vi "finish5RobotsPassGamePlay.vi"(8 "error in (no error)":errorcluster, 10 "Game in":refnum<class "Game.lvclass">, 11 "5RobotsPassGamePlay in":refnum<class "5RobotsPassGamePlay.lvclass">) -> (0 "error out":errorcluster, 1 "finish?":bool, 2 "Game out":refnum<class "Game.lvclass">, 3 "5RobotsPassGamePlay out":refnum<class "5RobotsPassGamePlay.lvclass">, 4 "debugOffensivePlayFinished":T1[](array[typedef]), 5 "degugBallVel":T2[](array[typedef]))   [LabVIEW 2020, in "5RobotsPassGamePlay.lvclass"]
uses:
  5RobotsPassGamePlay.lvclass
  C:/RoboIME/SSL_AI/Play_class/Play.lvclass
  Game_class/Game.lvclass
  PassFinishBallVelConditionDegub.ctl
  PassFinishReceiverDistanceToBallConditionDebug.ctl
  Referee_class/command_interpreted.ctl
  Utilities_class/Utilities.lvclass
  Robot_class/roles.ctl
  Game_class/Game.lvclass/Game.ctl
  Events_class/Events.lvclass/Events.ctl
  Object_class/Object.lvclass/Object.ctl
  Ball_class/Ball.lvclass/Ball.ctl
  Parameters_class/Parameters.lvclass/Parameters.ctl
  Referee_class/Referee.lvclass/Referee.ctl
  Team_class/Team.lvclass/Team.ctl
  Robot_class/Robot.lvclass/Robot.ctl
  Playbook_class/Playbook.lvclass/Playbook.ctl
  5RobotsPassGamePlay.lvclass/5RobotsPassGamePlay.ctl
  Playbook_class/Read offensive_plays.vi
  Write factorPassAlreadyCalculated_.vi
  Write passFinishConditions.vi
  Playbook_class/Write offensive_plays.vi
  Game_class/Read Parameters.lvclass.vi
  Parameters_class/Read BallVelToAbortPass.vi
  Parameters_class/Read minDistanceToPass.vi
  Game_class/Read EventsRef.vi
  Game_class/Read BallRef.vi
  Game_class/Read OffensiveTeam.vi
  Team_class/Read RobotRef.vi
  Team_class/Read OffensivePlay Finished.vi
  Object_class/Read x.vi
  Object_class/Read y.vi
  Robot_class/Read id.vi
  Ball_class/Read z.vi
  Ball_class/Read v_x.vi
  Ball_class/Read v_y.vi
  Events_class/Read touch.vi
  Events_class/Read enemy_ball_possesion.vi
  Events_class/Read id_touch.vi
  Events_class/Read ball_out.vi
  Game_class/Read Referee.vi
  Referee_class/Read command_interpreted.vi
  Ally_class/Ally.lvclass
  C:/RoboIME/SSL_AI/Team_class/Team.lvclass
  Robot_class/Robot.lvclass
  C:/RoboIME/SSL_AI/Object_class/Object.lvclass
  Ball_class/Ball.lvclass
  Referee_class/Referee.lvclass
  Events_class/Events.lvclass
  Parameters_class/Parameters.lvclass
  Playbook_class/Playbook.lvclass
  Play_class/Play.lvclass
  TestPlay_class/TestPlay.lvclass
  EnemyPossessionAtEnemyFieldPlay_class/EnemyPossessionAtEnemyFieldPlay.lvclass
  EnemyPossessionAtOurFieldPlay_class/EnemyPossessionAtOurFieldPlay.lvclass
  NormalGamePlay_class/NormalGamePlay.lvclass
  IndirectEnemyPlay_class/IndirectEnemyPlay.lvclass
  PrepareKickoffAllyPlay_class/PrepareKickoffAllyPlay.lvclass
  PrepareKickoffEnemyPlay_class/PrepareKickoffEnemyPlay.lvclass
  KickPenaltyAllyPlay_class/KickPenaltyAllyPlay.lvclass
  PreparePenaltyAllyPlay_class/PreparePenaltyAllyPlay.lvclass
  DirectEnemyPlay_class/DirectEnemyPlay.lvclass
  PreparePenaltyEnemyPlay_class/PreparePenaltyEnemyPlay.lvclass
  BallOutOfFieldPlay_class/BallOutOfFieldPlay.lvclass
  StopOffensivePlay_class/StopOffensivePlay.lvclass
  PassPlay_class/PassPlay.lvclass
  DirectKickPlay_class/DirectKickPlay.lvclass
  HaltPlay_class/HaltPlay.lvclass
  PreparePassPlay_class/PreparePassPlay.lvclass
  PassToStriker_class/PassToStriker.lvclass
  PassTo2ndStriker_class/PassTo2ndStriker.lvclass
  SimplePass_class/SimplePass.lvclass
  PrepareRollToPassPlay_class/PrepareRollToPassPlay.lvclass
  PrepareDoublePassPlay_class/PrepareDoublePassPlay.lvclass
  TableWith2ndStrikerPlay_class/TableWith2ndStrikerPlay.lvclass
  TableWithStrikerPlay_class/TableWithStrikerPlay.lvclass
  PrepareTriplePassPlay_class/PrepareTriplePassPlay.lvclass
  ABCPassPlay_class/ABCPassPlay.lvclass
  PreparePassInGame1_class/PreparePassInGame1.lvclass
  ACBPassPlay_class/ACBPassPlay.lvclass
  PrepareKeeperPassPlay_class/PrepareKeeperPassPlay.lvclass
  KeeperPassToStrikerPlay_class/KeeperPassToStrikerPlay.lvclass
  5RobotsNormalGamePlay_class/5RobotsNormalGamePlay.lvclass
  5RobotsKeeperGame_class/5RobotsKeeperGame.lvclass
panel:
  in  "ReceiverDistanceToBallConditionDebug":T1
  in  "BallVelConditionDebug":T2
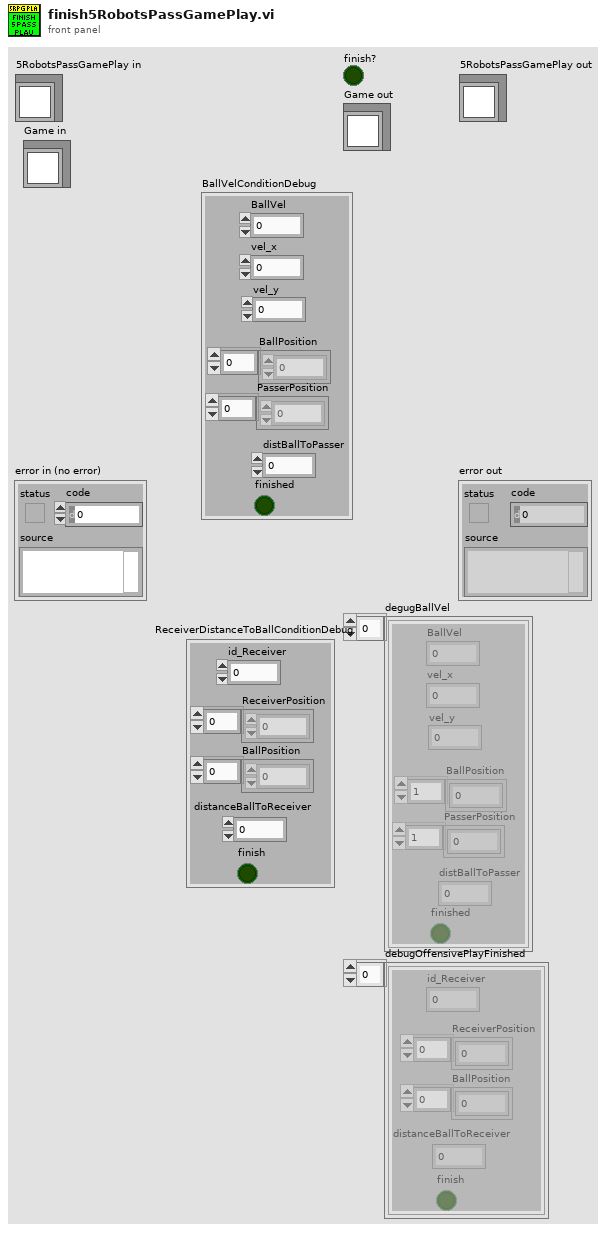
[diagram p1: front panel]
types:
  T1 = typedef "PassFinishReceiverDistanceToBallConditionDebug.ctl" = cluster{"id_Receiver":i32, "ReceiverPosition":dbl[], "BallPosition":dbl[], "distanceBallToReceiver":dbl, "finish":bool}
  T2 = typedef "PassFinishBallVelConditionDegub.ctl" = cluster{"BallVel":dbl, "BallPosition":dbl[], "PasserPosition":dbl[], "distBallToPasser":dbl, "finished":bool, "vel_x":dbl, "vel_y":dbl}
  T3 = typedef "roles.ctl" = enum16{"SecondMarker", "5Robots5th", "PassBestReceiver", "5Robots4th", "5Robots3rd", "5Robots2nd", "5Robots1st", "PassBestRobot", "WaitPass", "ABCThirdKicker", "ABCFirstKicker", "ABCSecondKicker", "Tabler", "TableFinalizer", "PrepareRollToPassRoller", "PrepareRollToPassReceiver", "SimplePassRoll", "SimplePassRollReceiver", "PenaltyDefense", "PreparePassReceiver 2", "PreparePassReceiver 1", "PassObserver", "Timeout", "Goto", "ZigZag", "None", "BallOutOfField", "DefenderArea", "Duelist", "AttackerStop", "FollowAttacker", "KeeperRole", "KickPenalty", "AttackerAimGoal", "AttackerBlock", "Marker", "Halt", "Shoot", "PassKicker", "PassReceiver", "TestRole", "PenaltyAttacker"}
  T4 = typedef "command_interpreted.ctl" = enum16{"Goal Ally", "Goal Enemy", "Ball Placement Enemy", "Ball Placement Ally", "Normal Half Time", "Extra Time  Break", "Extra Half Time", "None", "Post Game", "PKA Normal Start", "Prepare Kickoff Ally", "PKE Normal Start", "Prepare Kickoff Enemy", "Force Start", "Halt", "Timeout", "Prepare Penalty Ally", "Prepare Penalty Enemy", "PPA NormalStart", "PPE Normal Start", "Indirect Free Ally", "Direct Free Enemy", "Direct Free Ally", "Indirect Free Enemy", "Stop"}
  T5 = typedef "offensive_plays.ctl" = cluster{"Play":refnum<class "Play.lvclass">, "TestPlay":refnum<class "TestPlay.lvclass">, "EnemyPossessionAtEnemyFieldPlay":refnum<class "EnemyPossessionAtEnemyFieldPlay.lvclass">, "EnemyPossessionAtOurFieldPlay":refnum<class "EnemyPossessionAtOurFieldPlay.lvclass">, "NormalGamePlay":refnum<class "NormalGamePlay.lvclass">, "IndirectEnemyPlay":refnum<class "IndirectEnemyPlay.lvclass">, "PrepareKickoffAllyPlay":refnum<class "PrepareKickoffAllyPlay.lvclass">, "PrepareKickoffEnemyPlay":refnum<class "PrepareKickoffEnemyPlay.lvclass">, "KickPenaltyAllyPlay":refnum<class "KickPenaltyAllyPlay.lvclass">, "PreparePenaltyAllyPlay":refnum<class "PreparePenaltyAllyPlay.lvclass">, "DirectEnemyPlay":refnum<class "DirectEnemyPlay.lvclass">, "PreparePenaltyEnemyPlay":refnum<class "PreparePenaltyEnemyPlay.lvclass">, "BallOutOfFieldPlay":refnum<class "BallOutOfFieldPlay.lvclass">, "StopOffensivePlay":refnum<class "StopOffensivePlay.lvclass">, "PassPlay":refnum<class "PassPlay.lvclass">, "DirectKickPlay":refnum<class "DirectKickPlay.lvclass">, "HaltPlay":refnum<class "HaltPlay.lvclass">, "PreparePassPlay":refnum<class "PreparePassPlay.lvclass">, "PassToStrikerPlay":refnum<class "PassToStriker.lvclass">, "PassTo2ndStrikerPlay":refnum<class "PassTo2ndStriker.lvclass">, "SimplePassPlay":refnum<class "SimplePass.lvclass">, "PrepareRollToPassPlay":refnum<class "PrepareRollToPassPlay.lvclass">, "PrepareDoublePassPlay":refnum<class "PrepareDoublePassPlay.lvclass">, "TableWith2ndStrikerPlay":refnum<class "TableWith2ndStrikerPlay.lvclass">, "TableWithStrikerPlay":refnum<class "TableWithStrikerPlay.lvclass">, "PrepareTriplePassPlay":refnum<class "PrepareTriplePassPlay.lvclass">, "ABCPassPlay":refnum<class "ABCPassPlay.lvclass">, "PreparePassInGame1":refnum<class "PreparePassInGame1.lvclass">, "ACBPassPlay":refnum<class "ACBPassPlay.lvclass">, "PrepareKeeperPassPlay":refnum<class "PrepareKeeperPassPlay.lvclass">, "KeeperPassToStrikerPlay":refnum<class "KeeperPassToStrikerPlay.lvclass">, "SimplePass":refnum<class "SimplePass.lvclass">, "SimplePass 2":refnum<class "SimplePass.lvclass">, "5RobotsNormalGamePlay":refnum<class "5RobotsNormalGamePlay.lvclass">, "5RobotsPassGamePlay":refnum<class "5RobotsPassGamePlay.lvclass">, "5RobotsKeeperGame":refnum<class "5RobotsKeeperGame.lvclass">}
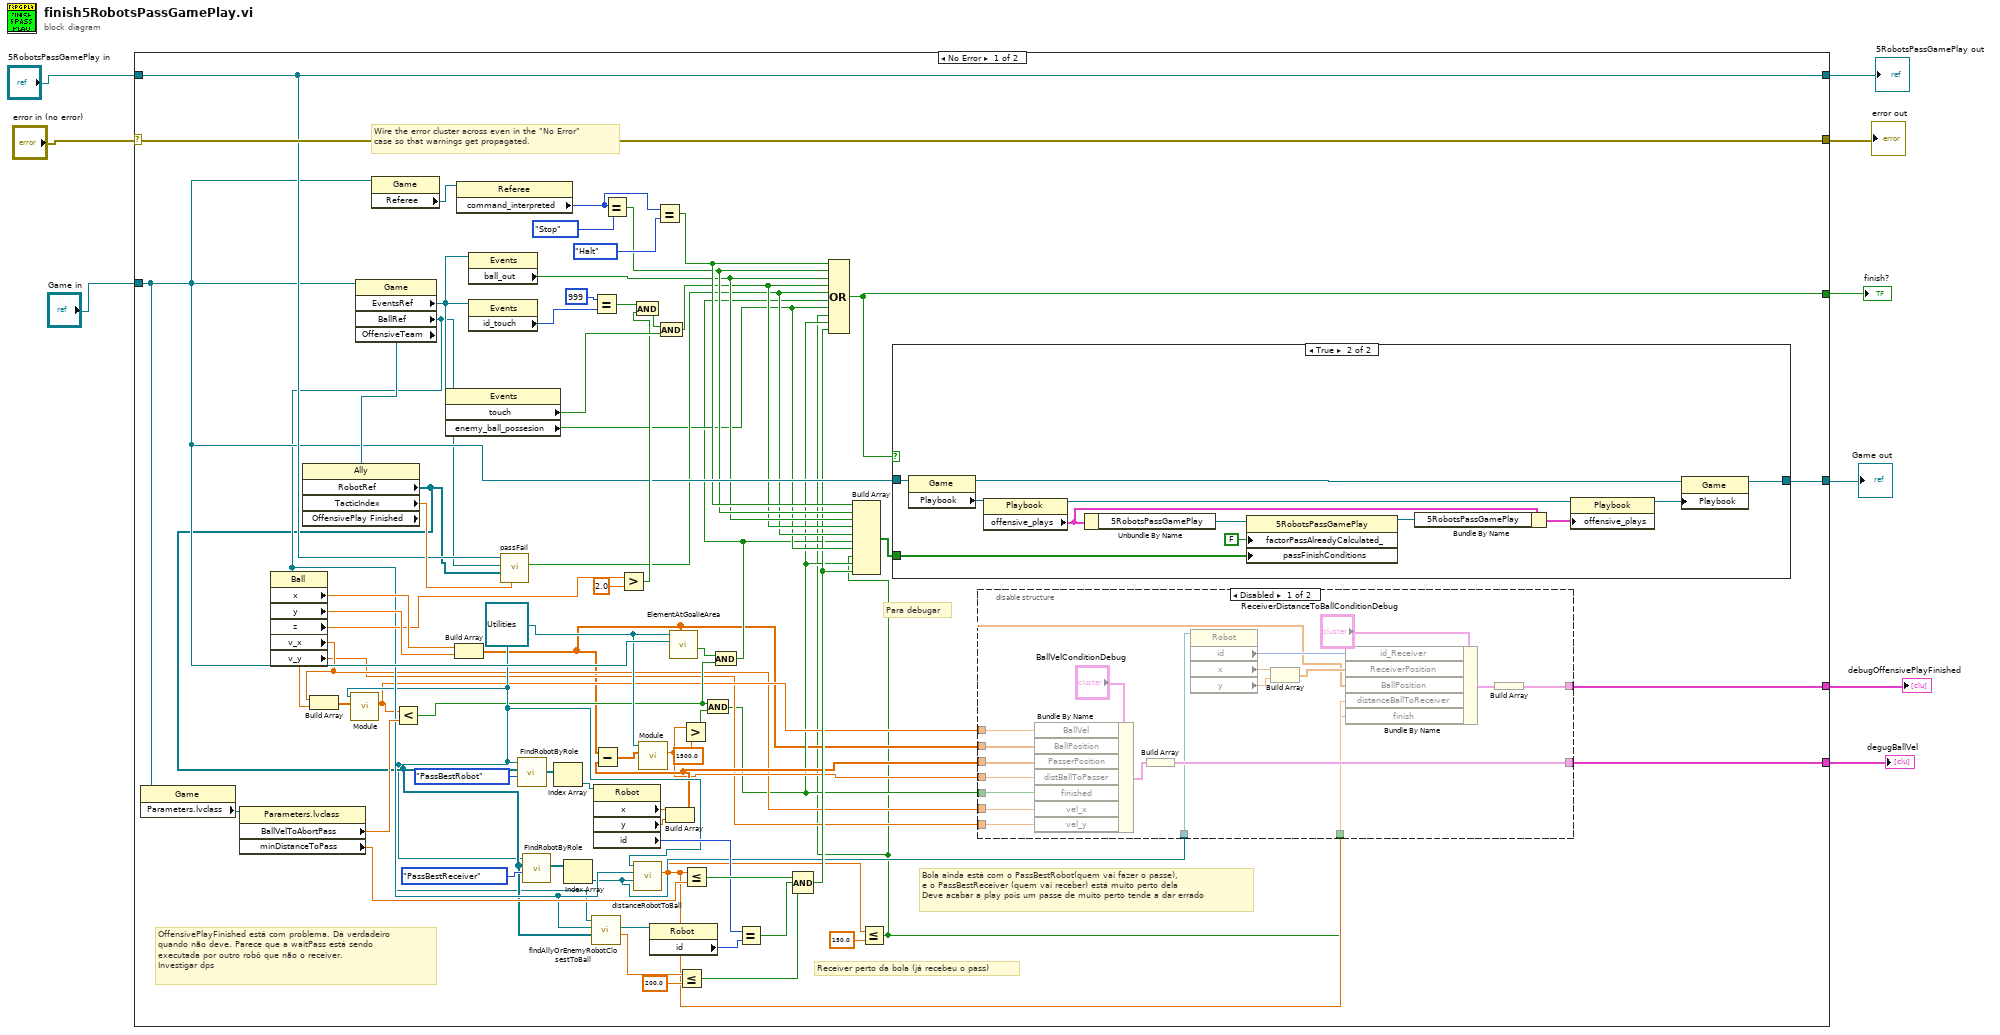
[diagram p0: block diagram]
diagram:
  n1 = case shown="No Error" "error in (no error)" {
    selector: "error in (no error)" -> [w80 w115]
    tunnel: [w80 w115] -> w4
    tunnel: [w62 w114] -> w8
    tunnel: "5RobotsPassGamePlay in" -> [w62 w114]
    tunnel: [w50 _] -> w6
    tunnel: "Game in" -> [w49 _]
    tunnel: [w48 _] -> w3
    tunnel: [w20 _] -> w2
    tunnel: [w13 _] -> w1
    frame No Error {
      w38 = refnum<class "Utilities.lvclass"> refnum ("Utilities in")
      # "Para debugar"
      # "Receiver perto da bola (já recebeu o pass)"
      # "OffensivePlayFinished está com problema. Dá verdadeiro\nquando não deve. Parece que a waitPass está sendo\nexecutada por outro robô que não o receiver.\nInvestigar dps"
      # "Bola ainda está com o PassBestRobot(quem vai fazer o passe),\ne o PassBestReceiver (quem vai receber) está muito perto dela\nDeve acabar a play pois um passe de muito perto tende a dar errado"
      # "Wire the error cluster across even in the \"No Error\"\ncase so that warnings get propagated."
      n2 = property class="Game"(reference=w49) -> ("Parameters.lvclass"=w52:refnum<class "Parameters.lvclass">)  [unwired: 1 in, 2 out]
      n3 = property class="Parameters.lvclass"(reference=w52) -> ("BallVelToAbortPass"=w51:dbl, "minDistanceToPass"=w45:dbl)  [unwired: 1 in, 2 out]
      n4 = property class="Game"(reference=w49) -> ("EventsRef"=w79:refnum<class "Events.lvclass">, "BallRef"=w42:refnum<class "Ball.lvclass">, "OffensiveTeam"=w71:refnum<class "Ally.lvclass">)  [unwired: 1 in, 2 out]
      n5 = property class="Ball"(reference=w42) -> ("x"=w70:dbl, "y"=w69:dbl, "z"=w67:dbl, "v_x"=w19:dbl, "v_y"=w18:dbl)  [unwired: 1 in, 2 out]
      n6 = property class="Ally" props=["RobotRef", "TacticIndex", "OffensivePlay Finished"](reference=w71) -> ("RobotRef"=w41:refnum<class "Robot.lvclass">[], "TacticIndex"=w68:dbl)  [unwired: 1 in, 3 out]
      n7 = Build Array(w19, w18) -> (w61:dbl[])
      n8 = call "Module.vi"("2D vector"=w61, "Utilities in"=w38) -> ("Modulo"=w23:dbl)  [unwired: 7 in, 2 out]
      n9 = property class="Game"(reference=w49) -> ("Referee"=w76:refnum<class "Referee.lvclass">)  [unwired: 1 in, 2 out]
      n10 = Less?(x=w23, y=w51) -> (x < y?=w25:bool)
      n11 = property class="Events"(reference=w79) -> ("touch"=w75:bool, "enemy_ball_possesion"=w29:bool)  [unwired: 1 in, 2 out]
      n12 = Build Array(w70, w69) -> (w14:dbl[])
      n13 = property class="Referee"(reference=w76) -> ("command_interpreted"=w73:T4)  [unwired: 1 in, 2 out]
      n14 = property class="Events"(reference=w79) -> ("ball_out"=w32:bool)  [unwired: 1 in, 2 out]
      n15 = property class="Events"(reference=w79) -> ("id_touch"=w77:i32)  [unwired: 1 in, 2 out]
      n16 = call "passFail.vi"("TacticIndex"=w68, "Offensive Robots"=w41, "Ball"=w42, "Play in"=w62) -> ("PassFail?"=w30:bool)  [unwired: 5 in, 2 out]
      n17 = call "FindRobotByRole.vi"("role"=roles."PassBestRobot", "RobotRef"=w41, "Utilities in"=w38) -> ("Robots"=w60:refnum<class "Robot.lvclass">[])  [unwired: 6 in, 2 out]
      n18 = call "FindRobotByRole.vi"("role"=roles."PassBestReceiver", "RobotRef"=w41, "Utilities in"=w38) -> ("Robots"=w46:refnum<class "Robot.lvclass">[])  [unwired: 6 in, 2 out]
      n19 = Index Array(array=w60) -> (element=w59:refnum<class "Robot.lvclass">)  [unwired: 1 in]
      n20 = Index Array(array=w46) -> (element=w15:refnum<class "Robot.lvclass">)  [unwired: 1 in]
      n21 = call "findAllyOrEnemyRobotClosestToBall.vi"("Ally/Enemy Robots"=w41, "Ball"=w42, "Utilities in"=w38) -> ("Robot distance to ball"=w37:dbl, "Robot"=w43:refnum<class "Robot.lvclass">)  [unwired: 5 in, 2 out]
      n22 = Equal?(x=999 ("id_touch"), y=w77) -> (x = y?=w65:bool)
      n23 = property class="Robot"(reference=w59) -> ("x"=w57:dbl, "y"=w56:dbl, "id"=w40:i32)  [unwired: 1 in, 2 out]
      n24 = Equal?(x=w73, y=command_interpreted."Stop") -> (x = y?=w33:bool)
      n25 = Greater?(x=w67, y=2.0) -> (0:w64:bool)
      n26 = And(x=w65, y=w64) -> (x .and. y?=w63:bool)
      n27 = call "distanceRobotToBall.vi"("Robot"=w15, "Ball"=w42, "Utilities in"=w38) -> ("Distance Robot To Ball"=w12:dbl)  [unwired: 6 in, 2 out]
      n28 = property class="Robot"(reference=w43) -> ("id"=w16:i32)  [unwired: 1 in, 2 out]
      n29 = Equal?(x=w73, y=command_interpreted."Halt") -> (x = y?=w34:bool)
      n30 = And(x=w63, y=w75) -> (x .and. y?=w31:bool)
      n31 = Build Array(w57, w56) -> (w22:dbl[])
      n32 = Subtract(x=w14, y=w22) -> (x-y=w55:dbl[])
      n33 = call "Module.vi"("2D vector"=w55, "Utilities in"=w38) -> ("Modulo"=w21:dbl)  [unwired: 7 in, 2 out]
      n34 = call-dynamic "ElementAtGoalieArea.vi"("Elemento pos."=w14, "Game"=w49, "Utilities in"=w38) -> ("Element at our goalkeeper area ?"=w26:bool)  [unwired: 5 in, 3 out]
      n35 = Less Or Equal?(x=w37, y=200.0) -> (x <= y?=w36:bool)
      n36 = Greater?(x=w21, y=1500.0) -> (0:w53:bool)
      n37 = Less Or Equal?(x=w12, y=w45) -> (x <= y?=w44:bool)
      n38 = And(x=w25, y=w53) -> (x .and. y?=w17:bool)
      n39 = And(x=w26, y=w25) -> (x .and. y?=w24:bool)
      n40 = Equal?(x=w40, y=w16) -> (x = y?=w39:bool)
      n41 = Compound Arithmetic op=AND(w44, w39, w36) -> (w28:bool)
      n42 = Less Or Equal?(x=w12, y=150.0) -> (x <= y?=w10:bool)
      n43 = Compound Arithmetic op=OR(w34, w33, w32, w31, w30, w24, w29, w10, w17, w28) -> (w50:bool)
      n44 = Build Array(w34, w33, w32, w31, w30, w24, w29, w10, w17, w28) -> (w27:bool[])
      n45 = case shown="True" w50 {
        tunnel: w49 -> [w101 w113]
        tunnel: [w101 w103] -> w48
        tunnel: w27 -> [_ w102]
        frame False {
        }
        frame True {
          n46 = property class="Game"(reference=w113) -> (reference out=w104:refnum<class "Game.lvclass">, "Playbook"=w112:refnum<class "Playbook.lvclass">)  [unwired: 1 in, 1 out]
          n47 = property class="Playbook"(reference=w112) -> (reference out=w106:refnum<class "Playbook.lvclass">, "offensive_plays"=w109:T5)  [unwired: 1 in, 1 out]
          n48 = Unbundle By Name(w109) -> ("5RobotsPassGamePlay"=w111:refnum<class "5RobotsPassGamePlay.lvclass">)
          n49 = property class="5RobotsPassGamePlay"(reference=w111, "factorPassAlreadyCalculated_"=FALSE, "passFinishConditions"=w102) -> (reference out=w108:refnum<class "5RobotsPassGamePlay.lvclass">)  [unwired: 1 in, 1 out]
          n50 = Bundle By Name(cluster=w109, "5RobotsPassGamePlay"=w108) -> (w107:T5)
          n51 = property class="Playbook"(reference=w106, "offensive_plays"=w107) -> (reference out=w105:refnum<class "Playbook.lvclass">)  [unwired: 1 in, 1 out]
          n52 = property class="Game"(reference=w104, "Playbook"=w105) -> (reference out=w103:refnum<class "Game.lvclass">)  [unwired: 1 in, 1 out]
        }
      }
      n53 = disable-structure shown="Disabled" {
        disable-tunnel: w23 -> [w99 _]
        disable-tunnel: w22 -> [w98 _]
        disable-tunnel: w21 -> [w97 _]
        disable-tunnel: [w95 _] -> w20
        disable-tunnel: w19 -> [w94 _]
        disable-tunnel: w18 -> [w93 _]
        disable-tunnel: w17 -> [w92 _]
        disable-tunnel: w15 -> [w90 _]
        disable-tunnel: w14 -> [w85 _]
        disable-tunnel: [w83 _] -> w13
        disable-tunnel: w12 -> [w82 _]
        disable-tunnel: w10 -> [w81 _]
        frame Disabled {
          n54 = Bundle By Name(cluster="BallVelConditionDebug", "BallVel"=w99, "BallPosition"=w85, "PasserPosition"=w98, "distBallToPasser"=w97, "finished"=w92, "vel_x"=w94, "vel_y"=w93) -> (w96:T2)
          n55 = Build Array(w96) -> (w95:T2[])
          n56 = property class="Robot"(reference=w90) -> ("id"=w89:i32, "x"=w88:dbl, "y"=w87:dbl)  [unwired: 1 in, 2 out]
          n57 = Build Array(w88, w87) -> (w86:dbl[])
          n58 = Bundle By Name(cluster="ReceiverDistanceToBallConditionDebug", "id_Receiver"=w89, "ReceiverPosition"=w86, "BallPosition"=w85, "distanceBallToReceiver"=w82, "finish"=w81) -> (w84:T1)
          n59 = Build Array(w84) -> (w83:T1[])
        }
        frame Enabled {
        }
      }
    }
    frame Error {
    }
  }
  "error out" <- w4
  "5RobotsPassGamePlay out" <- w8
  "finish?" <- w6
  "Game out" <- w3
  "degugBallVel" <- w2
  "debugOffensivePlayFinished" <- w1
